vi "剪切.vi"(8 "error in (no error)":errorcluster caption="错误输入（无错误）", 11 "程序 输入":refnum<class "程序.lvclass">) -> (0 "error out":errorcluster caption="错误输出", 3 "程序 输出":refnum<class "程序.lvclass">)   [LabVIEW 2018, in "程序.lvclass"]
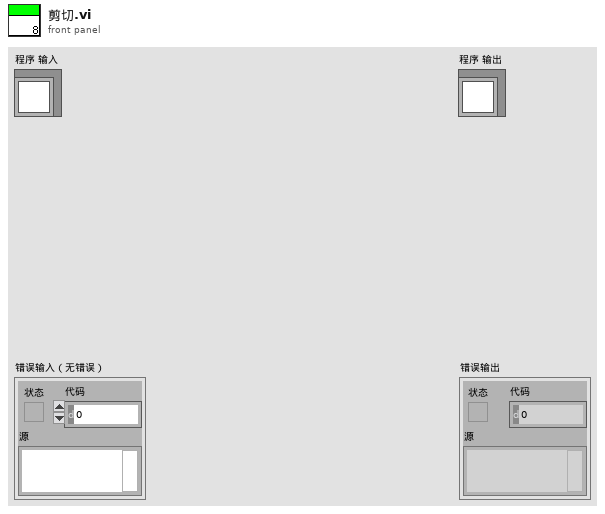
[diagram p1: front panel]
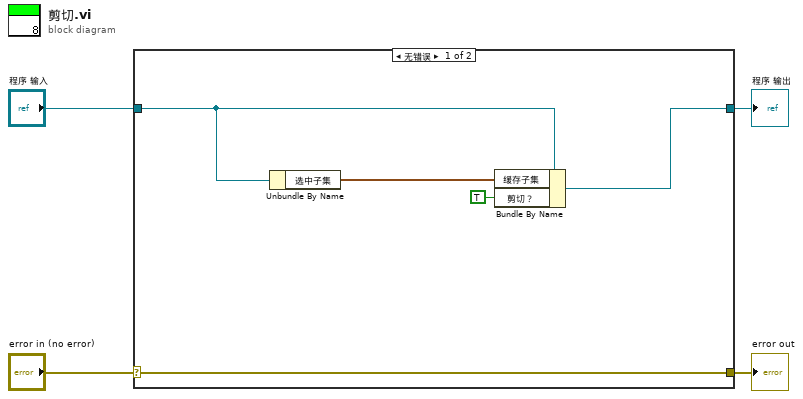
[diagram p0: block diagram]
diagram:
  n1 = case shown="无错误" "error in (no error)" {
    selector: "error in (no error)" -> [w9 w11]
    tunnel: [w9 w11] -> w3
    tunnel: [w5 w10] -> w1
    tunnel: "程序 输入" -> [w6 w10]
    frame No Error {
      n2 = Unbundle By Name(w6) -> ("选中子集"=w7:cluster{"行":i32, "列":i32}[])
      n3 = Bundle By Name(cluster=w6, "缓存子集"=w7, "剪切？"=TRUE) -> (w5:refnum<class "程序.lvclass">)
    }
    frame Error {
    }
  }
  "error out" <- w3
  "程序 输出" <- w1
